vi "Generic PC Build.vi"   [LabVIEW 2020]
uses:
  lv-builder/Builder Tools/Builder/Builder.lvclass
  lv-builder/Builder Tools/Simple Build GUI/Simple Build GUI.lvclass
panel:
  # "Generic PC Build"
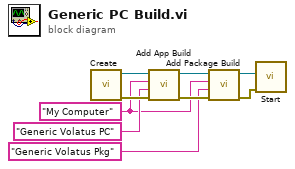
[diagram p0: block diagram]
diagram:
  w2 = "My Computer" ("Target")
  n1 = call "Create.vi"() -> ("error out"=w9:errorcluster, "Builder out"=w8:refnum<class "Builder.lvclass">)  [unwired: 10 in]
  n2 = call "Add App Build.vi"("error in (no error)"=w9, "Build Spec"="Generic Volatus PC" ("Target"), "Target"=w2, "Builder in"=w8) -> ("error out"=w6:errorcluster, "Builder out"=w4:refnum<class "Builder.lvclass">)  [unwired: 6 in]
  n3 = call "Add Package Build.vi"("error in (no error)"=w6, "Build Spec"="Generic Volatus Pkg" ("Target"), "Target"=w2, "Builder in"=w4) -> ("error out"=w5:errorcluster, "Builder out"=w3:refnum<class "Builder.lvclass">)  [unwired: 6 in]
  n4 = call "Start.vi"("error in (no error)"=w5, "Builder"=w3) -> ()  [unwired: 8 in, 2 out]
